vi "merFISH_ON_OFF_valve.vi"(2 "queue valve":refnum<queue>, 3 "error in":errorcluster, 4 "Valve on off":bool, 5 "Two-way Refnum":refnum<vi>) -> (0 "error out":errorcluster)   [LabVIEW 2015]
uses:
  CONTROLS/Q_VALVE_element.ctl
  GLOBAL/Global_ABORT.vi
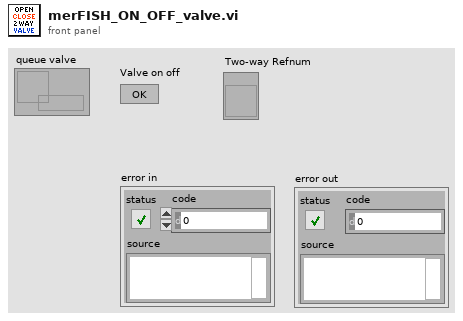
[diagram p1: front panel]
types:
  T1 = typedef "Q_VALVE_element.ctl" = cluster{"variant":variant, "Instruction":enum16{"VALVE_idle", "VALVE_initialize", "VALVE_error", "VALVE_security_stop", "VALVE_change_position", "VALVE_two_way_valves", "VALVE_init_merFISH", "VALVE_stop"}}
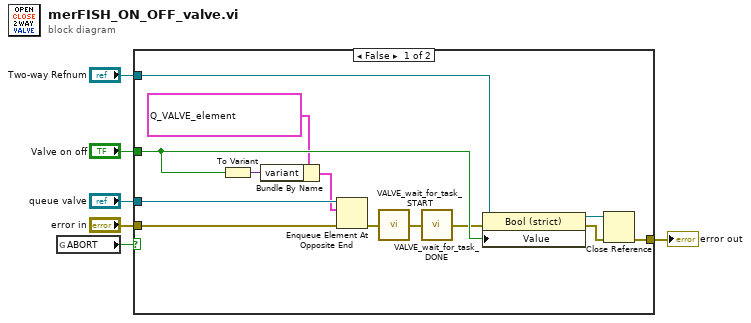
[diagram p0: block diagram]
diagram:
  n1 = global read "Global_ABORT.vi" "ABORT"() -> (w3:bool)
  n2 = case shown="False" w3 {
    tunnel: "queue valve" -> [w19 _]
    tunnel: "error in" -> [w18 w20]
    tunnel: "Two-way Refnum" -> [w16 _]
    tunnel: [w12 w20] -> w5
    tunnel: "Valve on off" -> [w15 _]
    frame False {
      n3 = To Variant(anything=w15) -> (Variant=w17:variant)
      n4 = Bundle By Name(cluster=T1 {"variant"=variant, "Instruction"=enum."VALVE_two_way_valves"} ("element"), "variant"=w17) -> (w10:T1)
      n5 = Enqueue Element At Opposite End(queue=w19, element=w10, error in (no error)=w18) -> (error out=w9:errorcluster)  [unwired: 1 in, 2 out]
      n6 = call "VALVE_wait_for_task_START.vi"("error in"=w9) -> ("error out"=w8:errorcluster)
      n7 = call "VALVE_wait_for_task_DONE.vi"("error in"=w8) -> ("error out"=w7:errorcluster)
      n8 = property class="Bool (strict)"(reference=w16, error in=w7, "Value"=w15) -> (reference out=w14:refnum<vi>, error out=w13:errorcluster)
      n9 = Close Reference(reference=w14, error in (no error)=w13) -> (error out=w12:errorcluster)
    }
    frame True {
    }
  }
  "error out" <- w5
